vi "Get cif_plugincore_FifoStatistics.vi"(8 "error in (no error)":errorcluster, 11 "gRPCid":T1) -> (0 "error out":errorcluster, 2 "package_templatemessage":T2, 3 "gRPCid out":T1)   [LabVIEW 2021, in "CIFCorePlugin_server.lvlib"]
uses:
  CIFCorePlugin_server.lvlib
  2ed25e12-861d-4677-8ead-ace2906b2041.vi
  cif_plugincore_TimingStatsBasic.ctl
  cif_plugincore_FifoStatistics.ctl
  cif_plugincore_TimingStatsBasic_Flat.ctl
  cif_plugincore_FifoStatistics_Flat.ctl
  <vilib>/gRPC/LabVIEW gRPC Library/Shared/grpcId.ctl
  <vilib>/gRPC/LabVIEW gRPC Library/grpc-lvsupport-release.lvlib
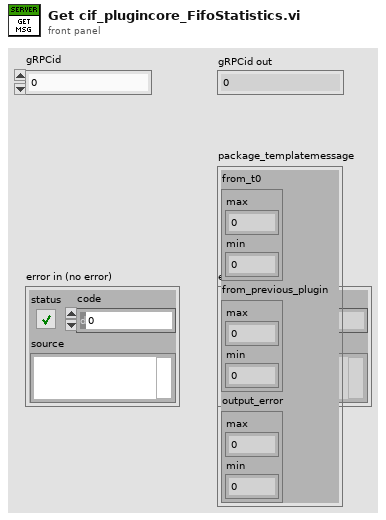
[diagram p1: front panel]
types:
  T1 = typedef "grpc-lvsupport-release.lvlib/grpcId.ctl" = u64
  T2 = typedef "CIFCorePlugin_server.lvlib/cif_plugincore_FifoStatistics.ctl" = cluster{"from_t0":T3, "from_previous_plugin":T3, "output_error":T3}
  T3 = typedef "CIFCorePlugin_server.lvlib/cif_plugincore_TimingStatsBasic.ctl" = cluster{"max":i32, "min":i32}
  T4 = typedef "CIFCorePlugin_server.lvlib/cif_plugincore_FifoStatistics_Flat.ctl" = cluster{"from_t0":T5, "from_previous_plugin":T5, "output_error":T5}
  T5 = typedef "CIFCorePlugin_server.lvlib/cif_plugincore_TimingStatsBasic_Flat.ctl" = cluster{"max":i32, "min":i32}
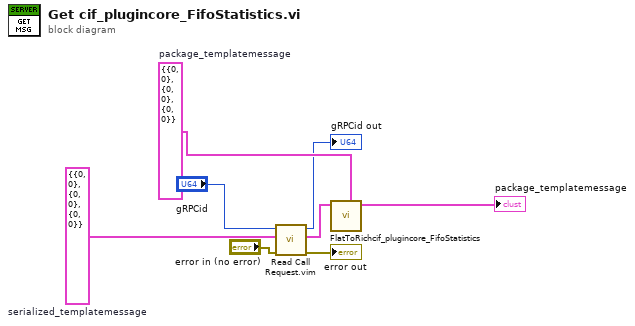
[diagram p0: block diagram]
diagram:
  w6 = T4 {"from_t0"={"max"=0, "min"=0}, "from_previous_plugin"={"max"=0, "min"=0}, "output_error"={"max"=0, "min"=0}}  # serialized_templatemessage
  w5 = T2 {"from_t0"={"max"=0, "min"=0}, "from_previous_plugin"={"max"=0, "min"=0}, "output_error"={"max"=0, "min"=0}}  # package_templatemessage
  n1 = call "Read Call Request.vim"("error in"="error in (no error)", "Request Type"=w6, "gRPCid in"="gRPCid") -> ("error out"=→"error out":errorcluster, "Request Data"=w4:T4, "gRPCid out"=→"gRPCid out":T1)  [unwired: 6 in]
  n2 = call "FlatToRichcif_plugincore_FifoStatistics.vi"("OutputClusterType"=w5, "InputCluster"=w4) -> ("OutputCluster"=→"package_templatemessage":T2)  [unwired: 9 in]
